vi "Get Scaling Factor.vi"(8 "error in (no error)":errorcluster, 11 "QRCodeDetector in":refnum<class "QRDetector.lvclass">) -> (0 "error out":errorcluster, 2 "Scale Factor":dbl, 3 "QRCodeDetector (Duplicate)":refnum<class "QRDetector.lvclass">)   [LabVIEW 2020, in "g_ar_toolkit.feature_detection.lvlib" / "QRDetector.lvclass"]
uses:
  QRDetector.lvclass
  QRDetector.lvclass/QRDetector.ctl
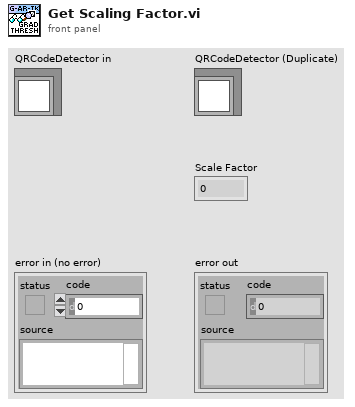
[diagram p1: front panel]
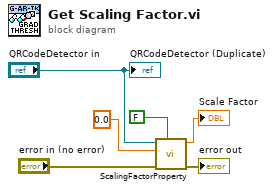
[diagram p0: block diagram]
diagram:
  n1 = call "ScalingFactorProperty.vi"("Write?"=FALSE, "error in (no error)"="error in (no error)", "Value in"=0.0 ("Value"), "QRCodeDetector in"="QRCodeDetector in") -> ("error out"=→"error out":errorcluster, "Value out"=→"Scale Factor":dbl)  [unwired: 6 in]
  "QRCodeDetector (Duplicate)" <- "QRCodeDetector in"
